vi "editDialog.vi"(0 "reference":refnum<class "InterfaceNode.lvclass">, 1 "insidePackageNode":bool, 5 "error in (no error)":errorcluster) -> (14 "reference out":refnum<class "InterfaceNode.lvclass">, 15 "changeConnection":T1, 16 "cancel":bool, 19 "error out":errorcluster)   [LabVIEW 2020, in "InterfaceNode.lvclass"]
doc: "Edit Dialog"
uses:
  <resource>/Framework/Providers/Open_GDS/UML/InterfaceNode_class/InterfaceNode.lvclass
  C:/Program Files (x86)/National Instruments/LabVIEW 2020/resource/Framework/Providers/Open_GDS/UML/AbstractNode_class/AbstractNode.lvclass
  <resource>/Framework/Providers/Open_GDS/UML/AbstractNode_class/private/NodeConnectionStatsType.ctl
  <resource>/Framework/Providers/Open_GDS/UML/ContextHelp/ContextHelp_HelpTexts.ctl
  <resource>/Framework/Providers/Open_GDS/UML/MultiLineString_class/MultiLineString.lvclass
  <resource>/Framework/Providers/Open_GDS/UML/AbstractNode_class/AbstractNode.lvclass
  <resource>/Framework/Providers/Open_GDS/UML/ClassNode_class/ClassNode.lvclass
panel:
  in  "Help":bool
  in  "AddMethod":bool
  in  "connection":bool caption="Connect to Package"
  in  "Class Name":string
  in  "Cancel Button":bool
  in  "OK Button":bool
  in  "Methods":string
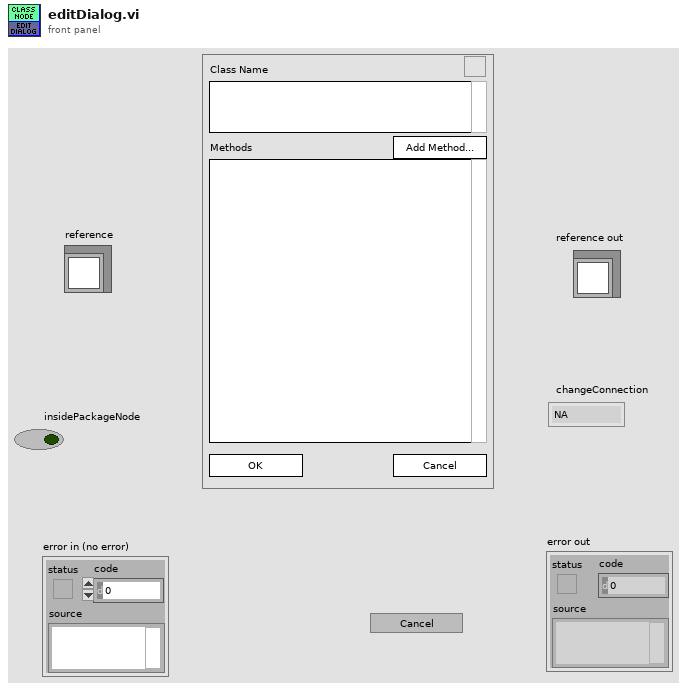
[diagram p1: front panel]
types:
  T1 = typedef "AbstractNode.lvclass/NodeConnectionStatsType.ctl" = enum16{"NA", "Connect", "DisConnect"}
  T2 = typedef "ContextHelp_HelpTexts.ctl" = enum16{"None(Hide)", "Default", "Help", "Welcome", "GettingStarted", "ClassDiagram_Help", "SequenceDiagram_Help", "UseCaseDiagram_Help", "BSelect", "BClass", "BInterface", "BPackage", "BNote", "BDependency", "BInheritance", "BInterfaceImplementation", "BAssociation", "BAggregation", "BCompAggregation", "BNoteConnector", "BObject", "BActionBar", "BCall", "BSystem", "BActor", "BUseCase", "BGeneralization", "BIncludes", "BExtends", "BUseCaseDiagramAssociation", "ClassRelationshipEdge editDialog_Bent Style", "ClassRelationshipEdge editDialog_RelationType", "ClassRelationshipEdge editDialog_Reverse association", "ClassRelationshipEdge editDialog_Start label", "ClassRelationshipEdge editDialog_Middle label", "ClassRelationshipEdge editDialog_End label", "UMLEditor reversedEngineering_Pathes", "ReversedEngineering StateReverseDialog_Help", "ReversedEngineering StateQueuedSettings_Help", "UMLEditor reversedEngineering_AddTopVIs", "UMLEditor reversedEngineering_AddClasses", "UMLEditor reversedEngineering_AddDirs", "UMLEditor reversedEngineering_Recursively", "UMLEditor reversedEngineering_Remove", "UMLEditor reversedEngineering_ClearList", "UMLEditor reversedEngineering_HideSubAss", "UMLEditor reversedEngineering_CreateTypes", "UMLEditor reversedEngineering_OnlyInheritance", "UMLEditor reversedEngineering_CreateApplication", "UMLEditor reversedEngineering_OK", "UMLEditor reversedEngineering_Cancel", "UMLEditor reversedEngineering_Help", "UMLEditor createWizardScriptFile_ScriptfilePath", "UMLEditor createWizardScriptFile_ClassPath", "UMLEditor createWizardScriptFile_Use", "UMLEditor createWizardScriptFile_PrivateDirName", "UMLEditor createWizardScriptFile_DirAppend", "UMLEditor createWizardScriptFile_Separator Character", "UMLEditor createWizardScriptFile_OK", "UMLEditor createWizardScriptFile_Cancel", "UMLEditor createWizardScriptFile_Help", "ClassNode editDialog_Class Name", "InterfaceNode editDialog_Class Name", "ClassNode editDialog_Attribute", "ClassNode editDialog_Methods", "InterfaceNode editDialog_Methods", "ClassNode editDialog_connection", "InterfaceNode editDialog_connection", "ClassNode editDialog_StereoType", "ClassNode editDialog_ShowAttrib", "ClassNode editDialog_ShowMethods", "ClassNode editDialog_ClassPath", "ClassNode editDialog_AddAttribute", "ClassNode editDialog_AddMethod", "InterfaceNode editDialog_AddMethod", "ClassNode AttributeGuide_AttributeName", "ClassNode AttributeGuide_Array?", "ClassNode AttributeGuide_Data Type", "ClassNode AttributeGuide_RefName", "ClassNode AttributeGuide_Preview", "ClassNode AttributeGuide_OK", "ClassNode AttributeGuide_Cancel", "ClassNode MethodGuide_Visibility", "ClassNode MethodGuide_Method Name", "ClassNode MethodGuide_Preview", "ClassNode MethodGuide_OK", "ClassNode MethodGuide_Cancel", "CallNode EditCallProperties_AllButtons", "ObjectNode EditObjectlProperties_AllButtons", "ActorNode EditActorProperties_AllButtons", "UseCaseRelationshipNode EditUseCaselProperties_AllButtons", "UseCaseNode EditUseCaselProperties_AllButtons", "SystemNode EditSystemProperties_AllButtons", "ReversedEngineering UpdateAttributes_AllButtons", "StateNode editDialog_AllButtons", "StateTransition editDialog_AllButtons", "ArrangeNodes Main_Picture", "ArrangeNodes Main_Zoom", "ArrangeNodes Main_Auto Zoom", "ArrangeNodes Main_shorten", "ArrangeNodes Main_Min Length", "ArrangeNodes Main_Max Length", "ArrangeNodes Main_increase", "ArrangeNodes Main_decrease", "ArrangeNodes Main_Shake", "ArrangeNodes Main", "BState", "BInitialState", "BFinalState", "BStateTransition", "StateDiagram_Help", "StateDiagram_PropertiesAllButtons", "ReversedEngineering StateReverseDialog_ClearStates", "ReversedEngineering StateReverseDialog_UseQueuedStateMachines", "ReversedEngineering StateReverseDialog_QueuedSettings", "ReversedEngineering StateReverseDialog_SearchForVIs", "ReversedEngineering StateReverseDialog_SearchCriteria", "OptionsDialog_ClassBasePath", "OptionsDialog_VIPath", "OptionsDialog_ApplicationPath", "OptionsDialog_WizDir", "OptionsDialog_IniFilePath", "OptionsDialog_DefineColors", "OptionsDialog_Help", "OptionsDialog_CreateTypes", "ClassRelationshipEdge editDialog_SplitWire"}
  T3 = typedef "InterfaceNode.lvclass/ObjectAttributes.ctl" = cluster{"midHeight":dbl, "botHeight":dbl, "name":refnum<class "MultiLineString.lvclass">, "methods":refnum<class "MultiLineString.lvclass">, "DEFAULT_COMPARTMENT_HEIGHT":i32, "DEFAULT_WIDTH":i32, "DEFAULT_HEIGHT":i32}
  T4 = typedef "AbstractNode.lvclass/ObjectAttributes.ctl" = cluster{"parent":refnum<class "AbstractNode.lvclass">, "children":refnum<class "AbstractNode.lvclass">[], "Hidden":bool}
  T5 = typedef "ContextHelp_ShowType.ctl" = cluster{"Header":string, "Picture":picture, "Text":string}
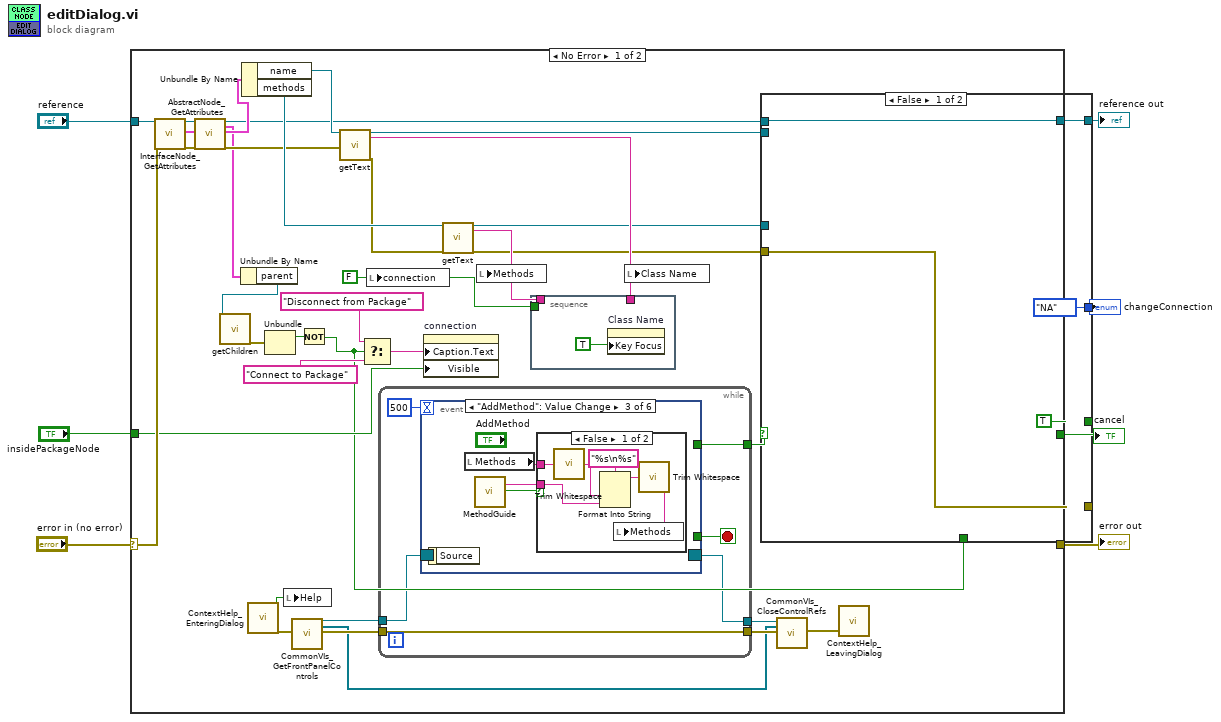
[diagram p0: block diagram]
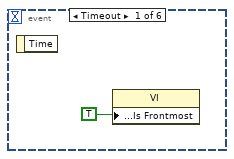
[diagram p2: hidden frame]
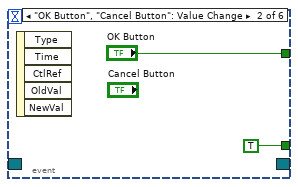
[diagram p3: hidden frame]
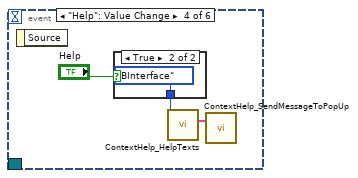
[diagram p5: hidden frame]
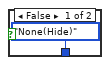
[diagram p6: hidden frame]
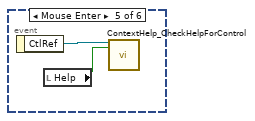
[diagram p7: hidden frame]
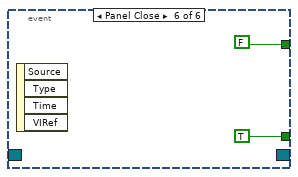
[diagram p8: hidden frame]
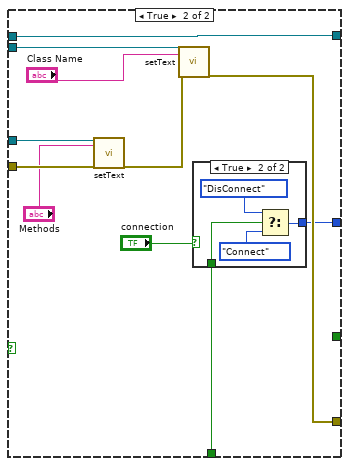
[diagram p9: hidden frame]
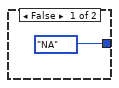
[diagram p10: hidden frame]
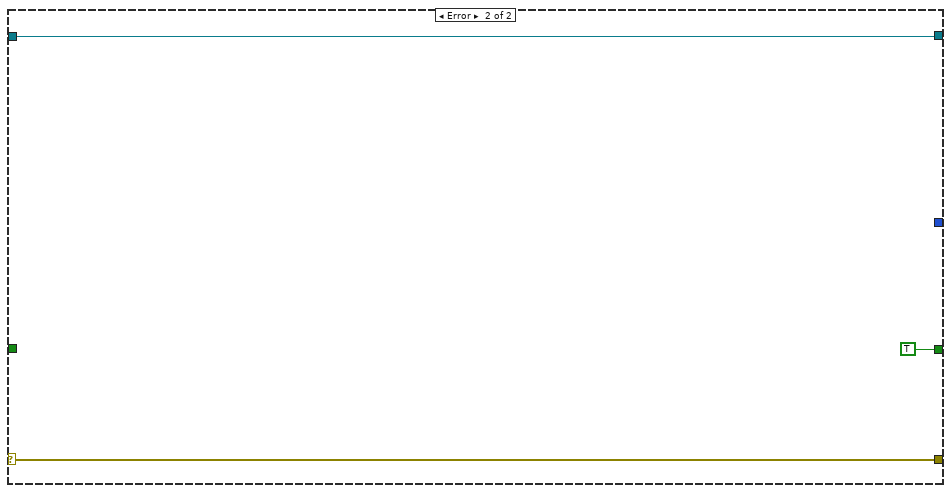
[diagram p11: hidden frame]
diagram:
  n1 = case shown="No Error" "error in (no error)" {
    selector: "error in (no error)" -> [w42 w95]
    tunnel: "reference" -> [w43 w96]
    tunnel: [w45 w95] -> w5
    tunnel: [w44 w96] -> w4
    tunnel: [w32 _] -> w3
    tunnel: "insidePackageNode" -> [w28 _]
    tunnel: [w26 TRUE ("Key Focus")] -> w1
    frame No Error {
      w27 = FALSE ("connection")
      n2 = call <resource>:"InterfaceNode_GetAttributes.vi"("reference in"=w43, "error in (no error)"=w42) -> ("reference out"=w12:refnum<class "InterfaceNode.lvclass">, "Data"=w13:T3, "error out"=w11:errorcluster)  [unwired: 1 in, 14 out]
      n3 = call <resource>:"AbstractNode_GetAttributes.vi"("reference in"=w12, "error in (no error)"=w11) -> ("reference out"=w9:refnum<class "InterfaceNode.lvclass">, "Data"=w8:T4, "error out"=w10:errorcluster)  [unwired: 14 in, 1 out]
      n4 = Unbundle By Name(w8) -> ("parent"=w15:refnum<class "AbstractNode.lvclass">)
      n5 = call-dynamic "getChildren.vi"("reference"=w15) -> ("error out"=w17:errorcluster)  [unwired: 15 in, 3 out]
      n6 = Unbundle By Name(w13) -> ("name"=w38:refnum<class "MultiLineString.lvclass">, "methods"=w36:refnum<class "MultiLineString.lvclass">)
      n7 = call <resource>:"ContextHelp_EnteringDialog.vi"() -> ("HelpStatus"=w23:bool, "error out"=w25:errorcluster)  [unwired: 3 in, 15 out]
      n8 = Unbundle(w17) -> ("status"=w16:bool)  [unwired: 2 out]
      n9 = local write "Help"(w23) -> ()
      n10 = call <resource>:"CommonVIs_GetFrontPanelControls.vi"("error in (no error)"=w25) -> ("Event Registration Refnum"=w19:refnum<event-registration>, "ControlRefs"=w20:refnum<vi>[], "error out"=w24:errorcluster)  [unwired: 1 in, 15 out]
      n11 = Not(x=w16) -> (.not. x?=w14:bool)
      n12 = call-dynamic "getText.vi"("reference"=w38, "error in (no error)"=w10) -> ("reference out"=w41:refnum<class "MultiLineString.lvclass">, "text"=w40:string, "error out"=w33:errorcluster)  [unwired: 15 in]
      n13 = Select(t="Disconnect from Package", s=w14, f="Connect to Package") -> (s? t:f=w31:string)
      n14 = local write "connection"(w27) -> ()
      n15 = while {
        tunnel: [w51] -> w39
        tunnel: [w48] -> w22
        tunnel: w24 -> [w48]
        tunnel: w19 -> [w47]
        tunnel: [w46] -> w18
        stop <- w49 stop-if-true
        n16 = event shown="[2] \"AddMethod\": Value Change" {
          selector: w47 -> [_ _ _ _ _ _]
          dyn-events: [_ _ _ _ _ _] -> w46
          timeout: 500 -> [_ _ _ _ _ _]
          tunnel: [_ "OK Button" _ _ _ FALSE ("OK Button")] -> w51
          tunnel: [_ TRUE _ _ _ TRUE ("Front Panel Window:Is Frontmost")] -> w49
          event Timeout {
            n17 = event-data() -> ()  [unwired: 2 out]
            n18 = property class="VI"("Front Panel Window:Is Frontmost"=TRUE) -> ()  [unwired: 2 in, 2 out]
          }
          event "OK Button", "Cancel Button": Value Change {
            n19 = event-data() -> ()  [unwired: 6 out]
          }
          event "AddMethod": Value Change {
            n20 = event-data() -> ()  [unwired: 2 out]
            n21 = local read "Methods"() -> (w57:string)
            n22 = call <resource>:"MethodGuide.vi"() -> ("Preview"=w56:string, "Canceled"=w55:bool)  [unwired: 1 in, 17 out]
            n23 = case shown="False" w55 {
              tunnel: w57 -> [w63 _]
              tunnel: w56 -> [w60 _]
              frame False {
                n24 = call <vilib>:"Trim Whitespace.vi"("string"=w63) -> ("trimmed string"=w61:string)  [unwired: 1 in]
                n25 = Format Into String(format string="%s\n%s", w61, w60) -> (resulting string=w59:string)  [unwired: 2 in, 1 out]
                n26 = call <vilib>:"Trim Whitespace.vi"("string"=w59) -> ("trimmed string"=w58:string)  [unwired: 1 in]
                n27 = local write "Methods"(w58) -> ()
              }
              frame True {
              }
            }
          }
          event "Help": Value Change {
            n28 = event-data() -> ()  [unwired: 2 out]
            n29 = case shown="True" "Help" {
              tunnel: [ContextHelp_HelpTexts."None(Hide)" ("HelpText") ContextHelp_HelpTexts."BInterface" ("HelpText")] -> w65
              frame False {
              }
              frame True {
              }
            }
            n30 = call <resource>:"ContextHelp_HelpTexts.vi"("HelpText (enum or string)"=w65) -> ("HelpOut"=w66:T5)  [unwired: 18 out]
            n31 = call <resource>:"ContextHelp_SendMessageToPopUp.vi"("PopUpMessage"=w66) -> ()  [unwired: 2 in, 17 out]
          }
          event Mouse Enter {
            n32 = event-data() -> ("CtlRef"=w70:refnum<vi>)  [unwired: 1 out]
            n33 = local read "Help"() -> (w69:bool)
            n34 = call <resource>:"ContextHelp_CheckHelpForControl.vi"("Ctl Refnum"=w70, "Help"=w69) -> ()  [unwired: 1 in, 17 out]
          }
          event Panel Close {
            n35 = event-data() -> ()  [unwired: 5 out]
          }
        }
      }
      n36 = property on="connection" class="Bool (strict)"("Caption.Text"=w31, "Visible"=w28) -> ()  [unwired: 2 in, 2 out]
      n37 = call-dynamic "getText.vi"("reference"=w36, "error in (no error)"=w33) -> ("reference out"=w35:refnum<class "MultiLineString.lvclass">, "text"=w37:string, "error out"=w34:errorcluster)  [unwired: 15 in]
      n38 = local write "Methods"(w37) -> ()
      n39 = stacked-sequence {
        tunnel: w40 -> [_]
        tunnel: w37 -> [_]
        tunnel: w27 -> [_]
        frame #0 {
          n40 = property on="Class Name" class="Str"("Key Focus"=TRUE) -> ()  [unwired: 2 in, 2 out]
        }
      }
      n41 = local write "Class Name"(w40) -> ()
      n42 = case shown="False" w39 {
        tunnel: [w75 w80] -> w45
        tunnel: [w76 w81] -> w44
        tunnel: w9 -> [w76 w81]
        tunnel: w41 -> [_ w87]
        tunnel: w35 -> [_ w86]
        tunnel: w34 -> [w75 w85]
        tunnel: [enum16{"NA", "Connect", "DisConnect"}."NA" ("changeConnection") w78] -> w32
        tunnel: w14 -> [_ w77]
        tunnel: [TRUE ("Key Focus") _] -> w26
        frame False {
        }
        frame True {
          n43 = call-dynamic "setText.vi"("reference"=w86, "text"="Methods", "error in (no error)"=w85) -> ("error out"=w82:errorcluster)  [unwired: 15 in, 1 out]
          n44 = call-dynamic "setText.vi"("reference"=w87, "text"="Class Name", "error in (no error)"=w82) -> ("error out"=w80:errorcluster)  [unwired: 15 in, 1 out]
          n45 = case shown="True" "connection" {
            tunnel: [enum16{"NA", "Connect", "DisConnect"}."NA" ("changeConnection") w91] -> w78
            tunnel: w77 -> [_ w92]
            frame False {
            }
            frame True {
              n46 = Select(t=enum16{"NA", "Connect", "DisConnect"}."DisConnect" ("changeConnection"), s=w92, f=enum16{"NA", "Connect", "DisConnect"}."Connect" ("changeConnection")) -> (s? t:f=w91:enum16{"NA", "Connect", "DisConnect"})
            }
          }
        }
      }
      n47 = call <resource>:"CommonVIs_CloseControlRefs.vi"("Event Registration Refnum"=w18, "ControlRefs"=w20, "error in (no error)"=w22) -> ("error out"=w21:errorcluster)  [unwired: 16 out]
      n48 = call <resource>:"ContextHelp_LeavingDialog.vi"("error in (no error)"=w21) -> ()  [unwired: 2 in, 17 out]
    }
    frame Error {
    }
  }
  "reference out" <- w4
  "error out" <- w5
  "changeConnection" <- w3
  "cancel" <- w1
